vi "LvIRKit_ManageDeviceData.vi"(7 "filepath":path=path "C:/EISOL/LvIRKIt/samples/sample.dat", 8 "action":T2(ring)=enum."Get", 9 "ip":string, 10 "name":string, 11 "id":i32) -> (1 "devdata out":T1, 2 "devdata[]":T3[](array[typedef]))   [LabVIEW 2014]
uses:
  LvIRKit_rsc_DeviceData_typedef.ctl
  LvIRKit_rsc_IRData_typedef.ctl
panel:
  out "size of devdata[]":i32
  in  "devdata":T3
  # "IP"
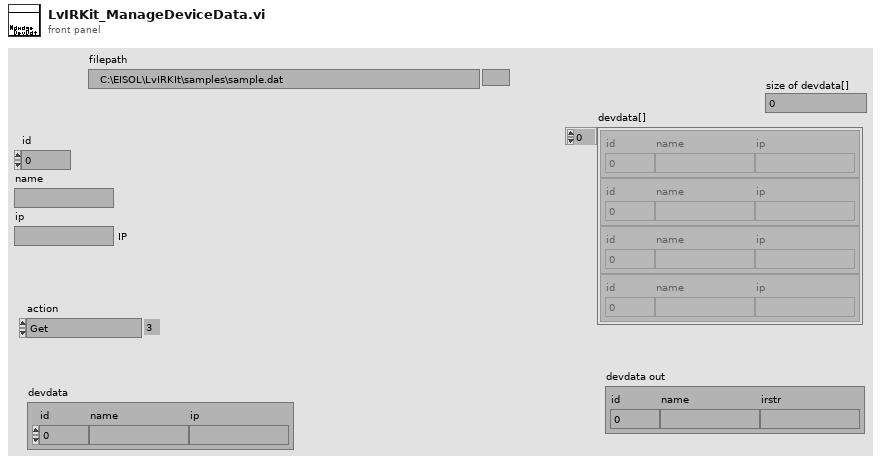
[diagram p1: front panel]
types:
  T1 = typedef "LvIRKit_rsc_IRData_typedef.ctl" = cluster{"id":i32, "name":string, "irstr":string}
  T2 = enum16{"Init", "Load", "Save", "Get", "Add", "Remove", "Replace", "Up", "Down"}
  T3 = typedef "LvIRKit_rsc_DeviceData_typedef.ctl" = cluster{"id":i32, "name":string, "ip":string}
  T4 = enum16{"open", "replace", "create", "open or create", "replace or create", "replace or create with confirmation"}
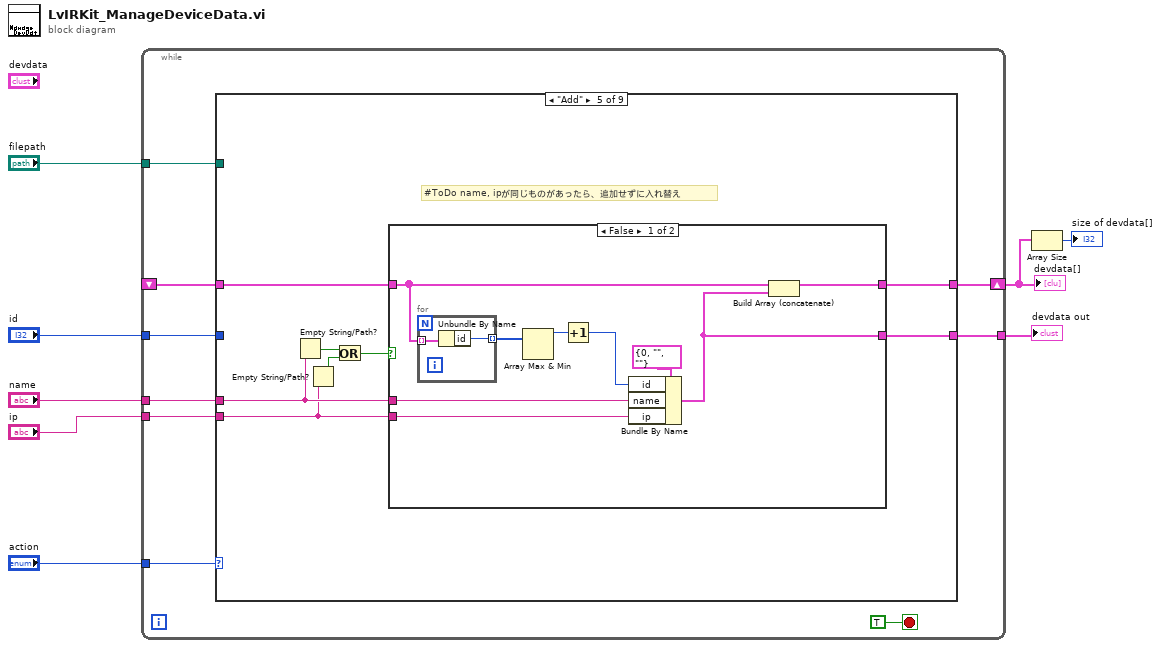
[diagram p0: block diagram]
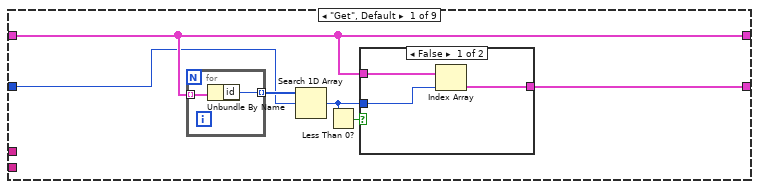
[diagram p2: hidden frame]
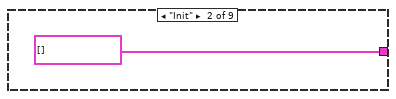
[diagram p4: hidden frame]
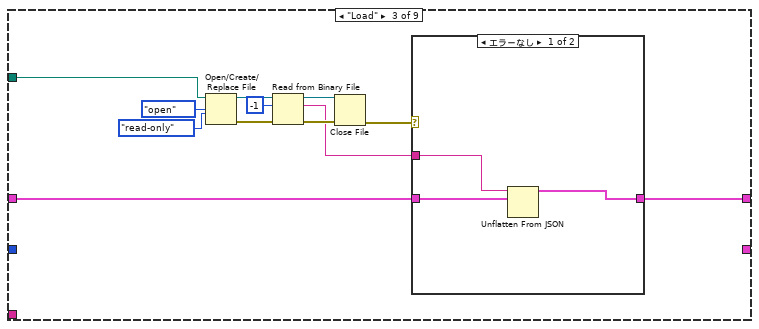
[diagram p5: hidden frame]
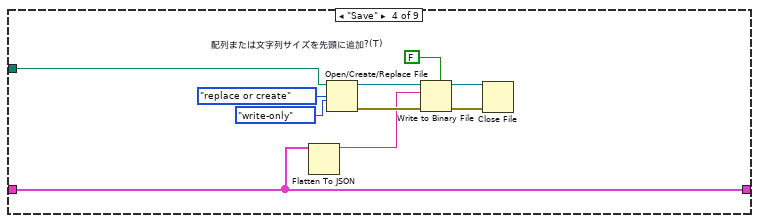
[diagram p7: hidden frame]
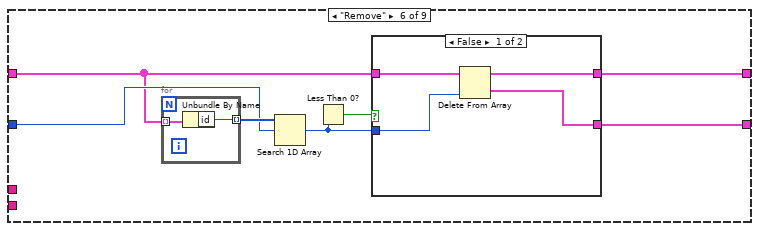
[diagram p9: hidden frame]
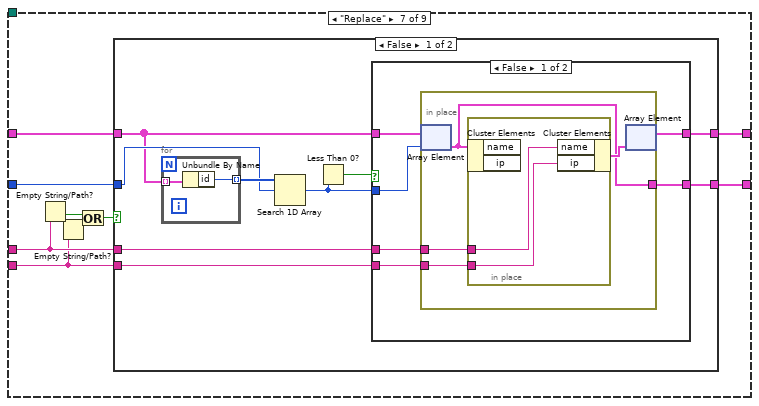
[diagram p11: hidden frame]
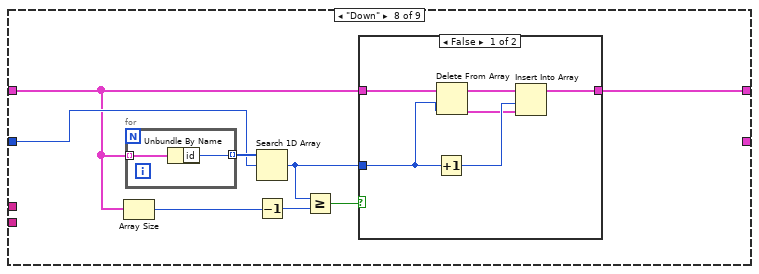
[diagram p14: hidden frame]
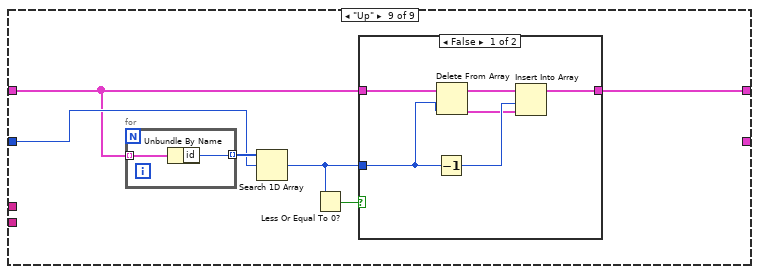
[diagram p16: hidden frame]
diagram:
  n1 = while {
    tunnel: "action" -> [w16]
    shift-right: [w15] -> w2
    shift-left: _ -> [w14]
    tunnel: "id" -> [w13]
    tunnel: [w12] -> w6
    tunnel: "name" -> [w11]
    tunnel: "ip" -> [w10]
    tunnel: "filepath" -> [w9]
    stop <- TRUE stop-if-true
    n2 = case shown="\"Add\"" w16 {
      tunnel: [w22 T1[] [] ("IRDATA[]") w32 w49 w63 w77 w96 w125 w143] -> w15
      tunnel: w14 -> [w22 _ w33 w49 w62 w78 w97 w126 w144]
      tunnel: w13 -> [w20 _ _ _ _ w81 w98 w130 w145]
      tunnel: [w23 _ _ _ w61 w76 w95 _ _] -> w12
      tunnel: w11 -> [_ _ _ _ w60 _ w94 _ _]
      tunnel: w10 -> [_ _ _ _ w59 _ w93 _ _]
      tunnel: w9 -> [_ _ w31 w46 _ _ _ _ _]
      frame "Get", Default {
        n3 = for {
          tunnel: w22 -> [w28] mode=indexing
          tunnel: [w27] -> w21 mode=indexing
          n4 = Unbundle By Name(w28) -> ("id"=w27:i32)
        }
        n5 = Search 1D Array(1D array=w21, element=w20) -> (index of element=w19:i32)  [unwired: 1 in]
        n6 = Less Than 0?(x=w19) -> (x < 0?=w18:bool)
        n7 = case shown="FALSE" w18 {
          tunnel: [w26 _] -> w23
          tunnel: w22 -> [w25 _]
          tunnel: w19 -> [w24 _]
          frame False {
            n8 = Index Array(array=w25, index=w24) -> (element=w26:T3)
          }
          frame True {
          }
        }
      }
      frame "Init" {
      }
      frame "Load" {
        n9 = Open/Create/Replace File(file path (use dialog)=w31, operation (0:open)=T4."open" ("操作（0:open）"), access (0:read/write)=enum16{"read/write", "read-only", "write-only"}."read-only" ("アクセス （0:read/write）")) -> (refnum out=w41:refnum<file>, error out=w40:errorcluster)  [unwired: 3 in, 1 out]
        n10 = Read from Binary File(8:w40, 10:-1 ("カウント（1）"), 11:w41) -> (0:w36:errorcluster, 2:w34:string, 3:w37:refnum<file>)  [unwired: 3 in, 1 out]
        n11 = Close File(refnum=w37, error in=w36) -> (error out=w35:errorcluster)  [unwired: 1 out]
        n12 = case shown="エラーなし" w35 {
          tunnel: w34 -> [w43 _]
          tunnel: w33 -> [w44 w45]
          tunnel: [w42 w45] -> w32
          frame No Error {
            n13 = Unflatten From JSON(JSON string=w43, type and defaults=w44) -> (value=w42:T3[])  [unwired: 5 in, 1 out]
          }
          frame Error {
          }
        }
      }
      frame "Save" {
        w47 = FALSE  # 配列または文字列サイズを先頭に追加?(T)
        n14 = Flatten To JSON(anything=w49) -> (JSON string=w48:string)  [unwired: 2 in, 1 out]
        n15 = Open/Create/Replace File(file path (use dialog)=w46, operation (0:open)=T4."replace or create" ("操作（0:open）"), access (0:read/write)=enum16{"read/write", "read-only", "write-only"}."write-only" ("アクセス （0:read/write）")) -> (refnum out=w55:refnum<file>, error out=w54:errorcluster)  [unwired: 3 in, 1 out]
        n16 = Write to Binary File(file (use dialog)=w55, data=w48, error in=w54, 5:w47) -> (refnum out=w51:refnum<file>, error out=w50:errorcluster)  [unwired: 2 in, 1 out]
        n17 = Close File(refnum=w51, error in=w50) -> ()  [unwired: 2 out]
      }
      frame "Add" {
        # "#ToDo name, ipが同じものがあったら、追加せずに入れ替え"
        n18 = Empty String/Path?(string/path=w60) -> (empty?=w58:bool)
        n19 = Empty String/Path?(string/path=w59) -> (empty?=w57:bool)
        n20 = Or(x=w58, y=w57) -> (x .or. y?=w56:bool)
        n21 = case shown="FALSE" w56 {
          tunnel: [w72 w75] -> w63
          tunnel: w60 -> [w71 _]
          tunnel: w59 -> [w70 _]
          tunnel: w62 -> [w69 w75]
          tunnel: [w65 _] -> w61
          frame False {
            n22 = for {
              tunnel: w69 -> [w74] mode=indexing
              tunnel: [w73] -> w68 mode=indexing
              n23 = Unbundle By Name(w74) -> ("id"=w73:i32)
            }
            n24 = Array Max & Min(array=w68) -> (max value=w67:i32)  [unwired: 3 out]
            n25 = Increment(x=w67) -> (x+1=w66:i32)
            n26 = Bundle By Name(cluster=T3 {"id"=0, "name"="", "ip"=""} ("devdata"), "id"=w66, "name"=w71, "ip"=w70) -> (w65:T3)
            n27 = Build Array (concatenate)(w69, w65) -> (w72:T3[])
          }
          frame True {
          }
        }
      }
      frame "Remove" {
        n28 = for {
          tunnel: w78 -> [w84] mode=indexing
          tunnel: [w83] -> w82 mode=indexing
          n29 = Unbundle By Name(w84) -> ("id"=w83:i32)
        }
        n30 = Search 1D Array(1D array=w82, element=w81) -> (index of element=w80:i32)  [unwired: 1 in]
        n31 = Less Than 0?(x=w80) -> (x < 0?=w79:bool)
        n32 = case shown="FALSE" w79 {
          tunnel: w80 -> [w86 _]
          tunnel: w78 -> [w88 w89]
          tunnel: [w87 w89] -> w77
          tunnel: [w85 _] -> w76
          frame False {
            n33 = Delete From Array(array=w88, index=w86) -> (deleted portion=w85:T3, array with subset deleted=w87:T3[])  [unwired: 1 in]
          }
          frame True {
          }
        }
      }
      frame "Replace" {
        n34 = Empty String/Path?(string/path=w94) -> (empty?=w92:bool)
        n35 = Empty String/Path?(string/path=w93) -> (empty?=w91:bool)
        n36 = Or(x=w92, y=w91) -> (x .or. y?=w90:bool)
        n37 = case shown="FALSE" w90 {
          tunnel: w98 -> [w106 _]
          tunnel: w97 -> [w103 w123]
          tunnel: [w102 w123] -> w96
          tunnel: [w101 _] -> w95
          tunnel: w94 -> [w100 _]
          tunnel: w93 -> [w99 _]
          frame False {
            n38 = for {
              tunnel: w103 -> [w109] mode=indexing
              tunnel: [w108] -> w107 mode=indexing
              n39 = Unbundle By Name(w109) -> ("id"=w108:i32)
            }
            n40 = Search 1D Array(1D array=w107, element=w106) -> (index of element=w105:i32)  [unwired: 1 in]
            n41 = Less Than 0?(x=w105) -> (x < 0?=w104:bool)
            n42 = case shown="FALSE" w104 {
              tunnel: w105 -> [w110 _]
              tunnel: w103 -> [w115 w122]
              tunnel: [w114 w122] -> w102
              tunnel: [w113 _] -> w101
              tunnel: w100 -> [w112 _]
              tunnel: w99 -> [w111 _]
              frame False {
                n43 = in-place {
                  in-place-border: [w116] -> w113
                  in-place-border: w112 -> [w118]
                  in-place-border: w111 -> [w117]
                  n44 = in-place-array #1(w115, w110) -> (w116:T3)
                  n45 = in-place {
                    in-place-border: w118 -> [w121]
                    in-place-border: w117 -> [w120]
                    n46 = in-place-cluster #2(w116) -> ()  [unwired: 2 out]
                    n47 = in-place-cluster #2("name"=w121, "ip"=w120) -> (w119:T3)
                  }
                  n48 = in-place-array #1(w119) -> (w114:T3[])  [unwired: 1 out]
                }
              }
              frame True {
              }
            }
          }
          frame True {
          }
        }
      }
      frame "Down" {
        n49 = Array Size(array=w126) -> (size(s)=w129:i32)
        n50 = for {
          tunnel: w126 -> [w140] mode=indexing
          tunnel: [w139] -> w131 mode=indexing
          n51 = Unbundle By Name(w140) -> ("id"=w139:i32)
        }
        n52 = Search 1D Array(1D array=w131, element=w130) -> (index of element=w124:i32)  [unwired: 1 in]
        n53 = Decrement(x=w129) -> (x-1=w128:i32)
        n54 = Greater Or Equal?(x=w124, y=w128) -> (x >= y?=w127:bool)
        n55 = case shown="FALSE" w127 {
          tunnel: w126 -> [w137 w138]
          tunnel: [w135 w138] -> w125
          tunnel: w124 -> [w134 _]
          frame False {
            n56 = Increment(x=w134) -> (x+1=w133:i32)
            n57 = Delete From Array(array=w137, index=w134) -> (deleted portion=w132:T3, array with subset deleted=w136:T3[])  [unwired: 1 in]
            n58 = Insert Into Array(array=w136, index=w133, new element=w132) -> (w135:T3[])
          }
          frame True {
          }
        }
      }
      frame "Up" {
        n59 = for {
          tunnel: w144 -> [w155] mode=indexing
          tunnel: [w154] -> w146 mode=indexing
          n60 = Unbundle By Name(w155) -> ("id"=w154:i32)
        }
        n61 = Search 1D Array(1D array=w146, element=w145) -> (index of element=w142:i32)  [unwired: 1 in]
        n62 = Less Or Equal To 0?(x=w142) -> (x <= 0?=w141:bool)
        n63 = case shown="FALSE" w141 {
          tunnel: w144 -> [w152 w153]
          tunnel: [w150 w153] -> w143
          tunnel: w142 -> [w149 _]
          frame False {
            n64 = Decrement(x=w149) -> (x-1=w148:i32)
            n65 = Delete From Array(array=w152, index=w149) -> (deleted portion=w147:T3, array with subset deleted=w151:T3[])  [unwired: 1 in]
            n66 = Insert Into Array(array=w151, index=w148, new element=w147) -> (w150:T3[])
          }
          frame True {
          }
        }
      }
    }
  }
  "devdata[]" <- w2
  "devdata out" <- w6
  n67 = Array Size(array=w2) -> (size(s)=→"size of devdata[]":i32)
